vi "Hipot_Close.vi"(8 "Error In":errorcluster, 10 "PORT":string, 11 "Limit":string) -> (0 "error out":errorcluster, 2 "Result":bool, 3 "Data":string)   [LabVIEW 2013]
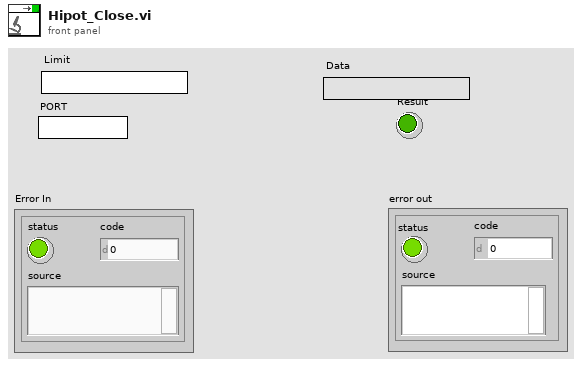
[diagram p1: front panel]
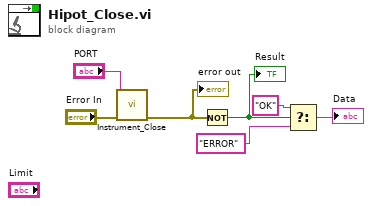
[diagram p0: block diagram]
diagram:
  n1 = call "Instrument_Close.vi"("Error In"="Error In", "PORT"="PORT") -> ("Error Out"=w2:errorcluster)  [unwired: 9 in]
  "error out" <- w2
  n2 = Not(x=w2) -> (.not. x?=w4:bool)
  "Result" <- w4
  n3 = Select(t="OK", s=w4, f="ERROR") -> (s? t:f=→"Data":string)
